vi "Handle getAll.vi"(8 "error in (no error)":errorcluster, 11 "Inst.Attocube-3DR in":refnum<class "Inst.Attocube-3DR.lvclass">) -> (0 "error out":errorcluster, 2 "getAll":variant, 3 "Inst.Attocube-3DR out":refnum<class "Inst.Attocube-3DR.lvclass">)   [LabVIEW 2019, in "Inst.Attocube-3DR.lvclass"]
uses:
  Inst.Attocube-3DR.lvclass
  Typedefs/Inst.Attocube-3DR.getAll--Cluster.ctl
  Inst.Attocube-3DR.lvclass/Inst.Attocube-3DR.ctl
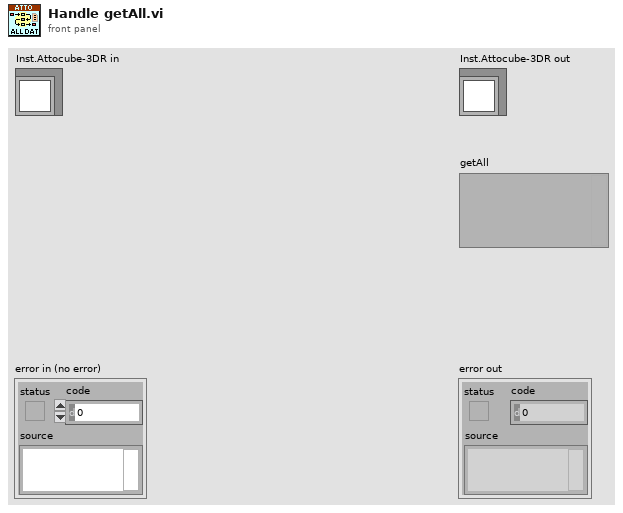
[diagram p1: front panel]
types:
  T1 = typedef "Inst.Attocube-3DR.lvclass/Inst.Attocube-3DR.getAll--Cluster.ctl" = cluster{"Levy 1":dbl, "Logger SMO":dbl, "SMO Boolean":bool, "SMO String":string}
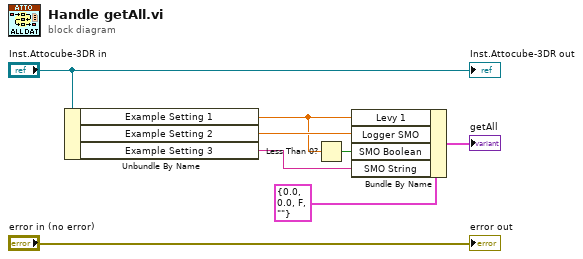
[diagram p0: block diagram]
diagram:
  n1 = Unbundle By Name("Inst.Attocube-3DR in") -> ("Example Setting 1"=w1:dbl, "Example Setting 2"=w4:dbl, "Example Setting 3"=w3:string)
  n2 = Less Than 0?(x=w1) -> (x < 0?=w2:bool)
  n3 = Bundle By Name(cluster=T1 {"Levy 1"=0.0, "Logger SMO"=0.0, "SMO Boolean"=FALSE, "SMO String"=""} ("getAll"), "Levy 1"=w1, "Logger SMO"=w4, "SMO Boolean"=w2, "SMO String"=w3) -> (→"getAll":T1)
  "error out" <- "error in (no error)"
  "Inst.Attocube-3DR out" <- "Inst.Attocube-3DR in"
